vi "Add Line.vi"(8 "error in":errorcluster, 10 "Line":T1, 11 "tag bus configurable plugin module configuration in":refnum<class "tag bus configurable plugin module configuration.lvclass">) -> (0 "error out":errorcluster, 3 "tag bus configurable plugin module configuration out":refnum<class "tag bus configurable plugin module configuration.lvclass">)   [LabVIEW 2014, in "tag bus configurable plugin module configuration.lvclass"]
uses:
  tag bus configurable plugin module configuration.lvclass
  Line.ctl
  <vilib>/NI/Tag Bus Module Framework/channel/TBM channel.lvclass
  tag bus configurable plugin module configuration.lvclass/tag bus configurable plugin module configuration.ctl
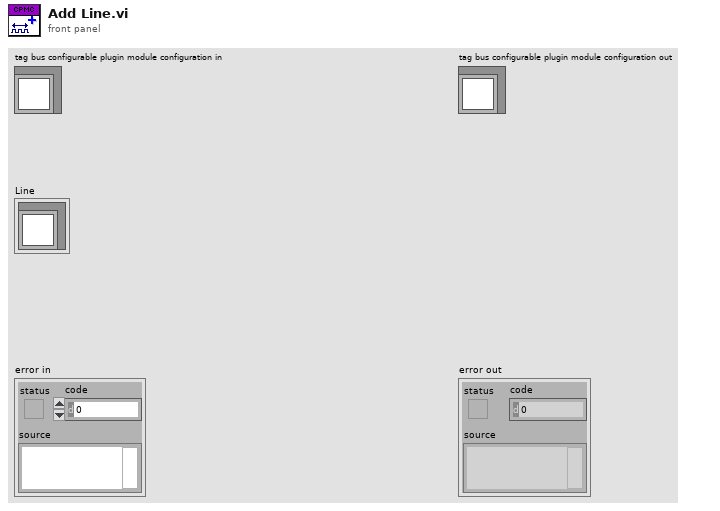
[diagram p1: front panel]
types:
  T1 = typedef "tag bus configurable plugin module configuration.lvclass/Line.ctl" = cluster{"channel":refnum<class "TBM channel.lvclass">}
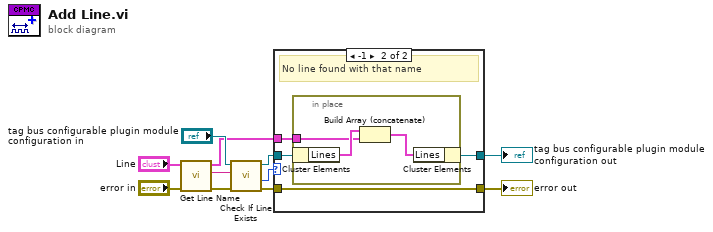
[diagram p0: block diagram]
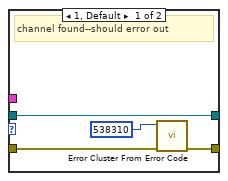
[diagram p2: hidden frame]
diagram:
  n1 = call "Get Line Name.vi"("error in"="error in", "Line in"="Line") -> ("error out"=w6:errorcluster, "Name"=w5:string, "Line out"=w3:T1)  [unwired: 7 in]
  n2 = call-dynamic "Check If Line Exists.vi"("error in"=w6, "name to locate"=w5, "tag bus configurable plugin module configuration in"="tag bus configurable plugin module configuration in") -> ("error out"=w7:errorcluster, "index"=w2:i32, "tag bus configurable plugin module configuration out"=w1:refnum<class "tag bus configurable plugin module configuration.lvclass">)  [unwired: 4 in, 2 out]
  n3 = case shown="-1" w2 {
    tunnel: [w15 w18] -> w11
    tunnel: w7 -> [w13 w18]
    tunnel: w1 -> [w12 w17]
    tunnel: w3 -> [_ w19]
    tunnel: [w12 w16] -> w10
    frame 1, Default {
      # "channel found--should error out"
      n4 = call <vilib>:"Error Cluster From Error Code.vi"("error in (no error)"=w13, "error code (0)"=538310) -> ("error out"=w15:errorcluster)  [unwired: 7 in]
    }
    frame -1 {
      # "No line found with that name"
      n5 = in-place {
        in-place-border: w19 -> [w20]
        n6 = in-place-cluster #1(w17) -> ("Lines"=w21:T1[])
        n7 = Build Array (concatenate)(w21, w20) -> (w22:T1[])
        n8 = in-place-cluster #1("Lines"=w22) -> (w16:refnum<class "tag bus configurable plugin module configuration.lvclass">)
      }
    }
  }
  "error out" <- w11
  "tag bus configurable plugin module configuration out" <- w10
